vi "Digital display.vi"() -> ()   [LabVIEW 2019]
uses:
  <vilib>/addons/Modulation/Analog/controls/Complex Data Waveform.ctl
  <vilib>/measure/madcrms.llb/Averaged DC-RMS for 1 Chan.vi
  <vilib>/addons/Modulation/niAMT.lvlib
  <vilib>/measure/NI_MAPro.lvlib
panel:
  out "Waveform Graph 5":waveform(dbl)(graph)
  out "Waveform Graph 4":waveform(dbl)(graph)
  out "Digital Waveform Graph 2":digitalwaveform(graph)
  out "Digital Waveform Graph":digitalwaveform(graph)
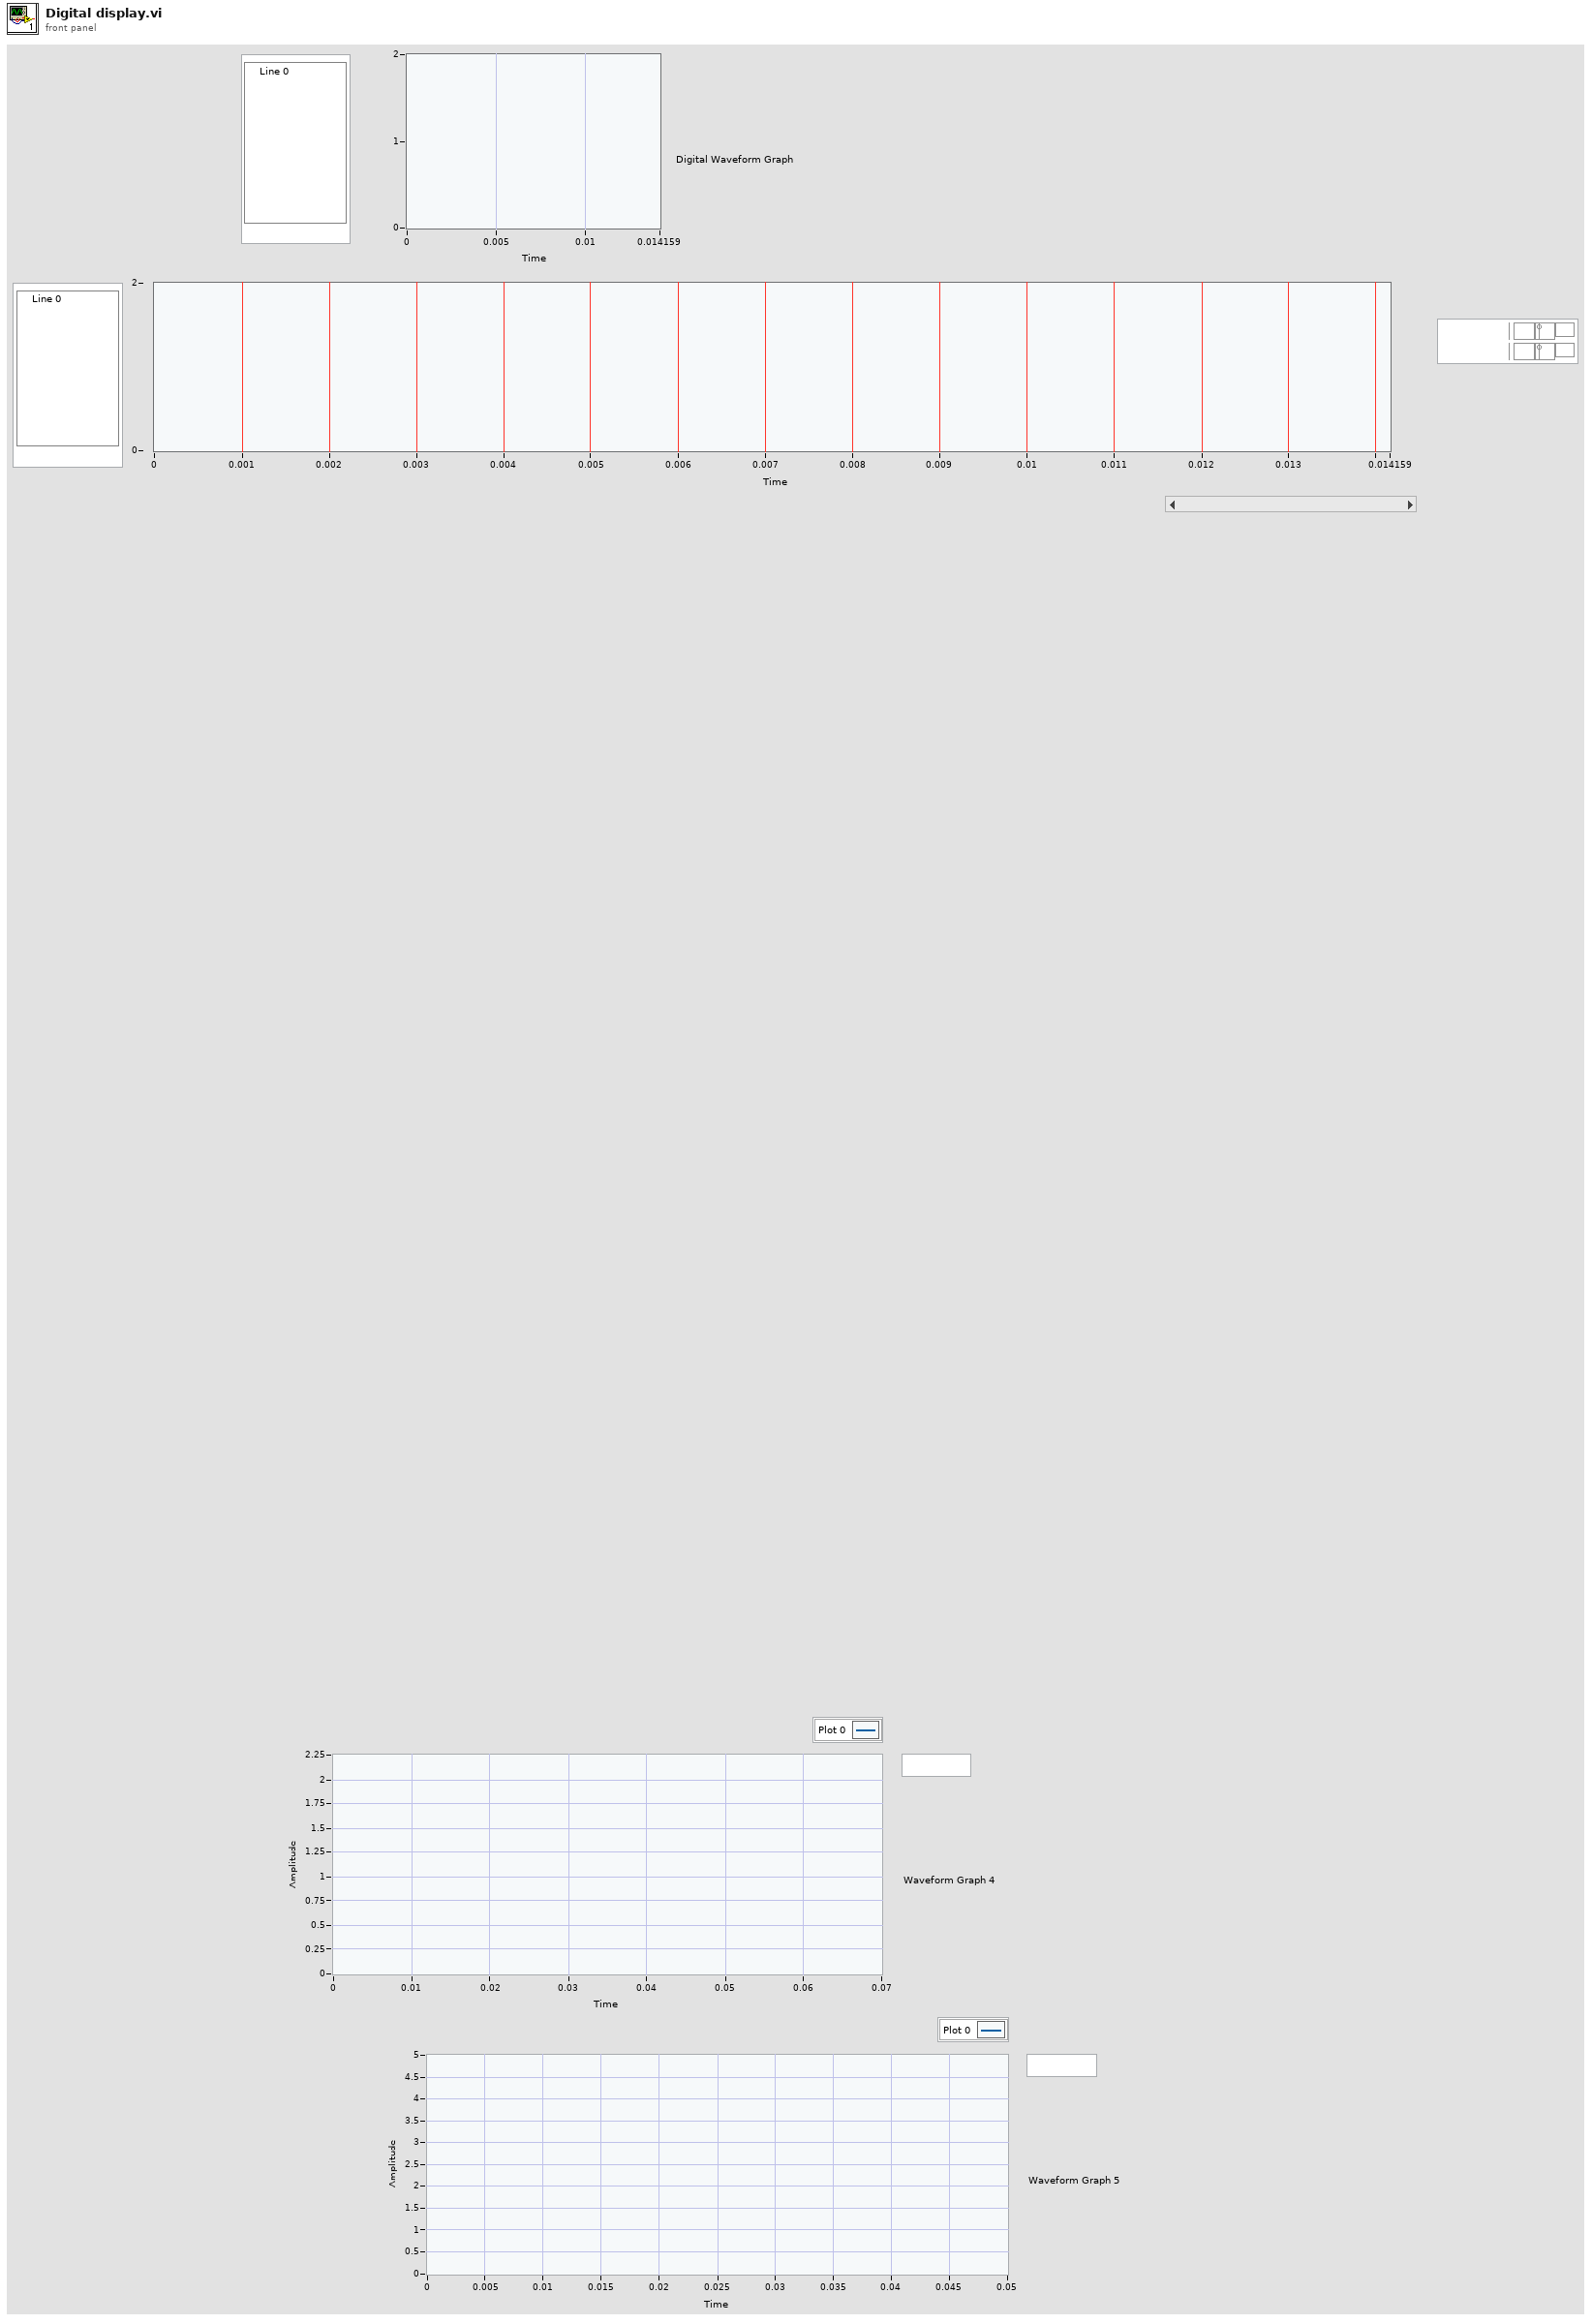
[diagram p1: front panel]
types:
  T1 = cluster{"window for DC":enum16{"Rectangular (none)", "Hanning", "Low side lobe"}, "output function":enum16{"DC only", "RMS only", "DC and RMS"}, "window for RMS":enum16{"Rectangular (none)", "Hanning", "Low side lobe"}, "exp. time constant":dbl, "Ignore input start time":bool}
  T2 = typedef "niAMT.lvlib/Complex Data Waveform.ctl" = cluster{"t0":dbl, "dt":dbl, "Y":cdb[]}
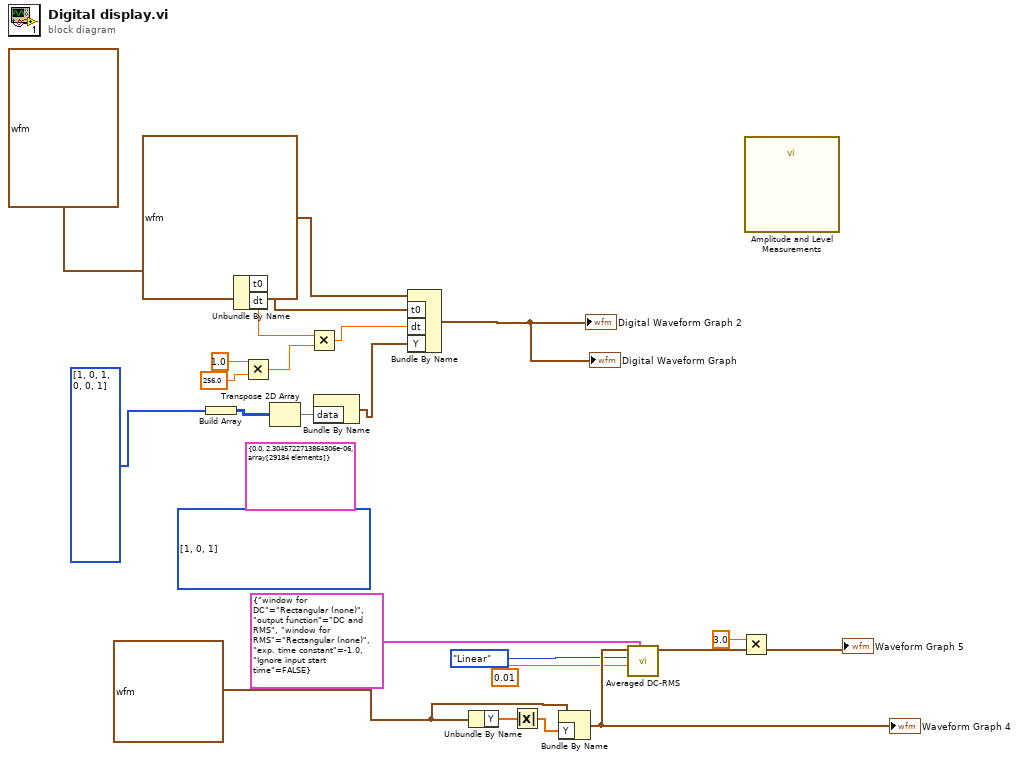
[diagram p0: block diagram]
diagram:
  w9 = waveform(dbl) {"t0"=timestamp(0 s since 1904-01-01), "dt"=2.3045722713864306e-06, "Y"=array[29568 elements]} ("Waveform out")
  (unwired) T2 {"t0"=0.0, "dt"=2.3045722713864306e-06, "Y"=array[29184 elements]} ("recovered complex waveform")
  (unwired) u8[][] [[1], [0], [1]] ("data")
  n1 = Build Array(i32[] [1, 0, 1, 0, 0, 1]) -> (w23:i32[][])
  n2 = Unbundle By Name(waveform(dbl) {"t0"=timestamp(6.868436578171096 s since 1904-01-01), "dt"=9.218289085545723e-06, "Y"=array[7296 elements]} ("Waveform")) -> ("t0"=w18:timestamp, "dt"=w17:dbl)
  n3 = Multiply(x=1.0 ("y"), y=256.0) -> (x*y=w13:dbl)
  n4 = Transpose 2D Array(2D array=w23) -> (transposed array=w21:i32[][])
  n5 = Multiply(x=w17, y=w13) -> (x*y=w16:dbl)
  n6 = Bundle By Name("data"=w21) -> (w20:digitaldata)  [unwired: 1 in]
  n7 = Bundle By Name(cluster=digitalwaveform {"t0"=timestamp(0 s since 1904-01-01), "dt"=1.0, "Y"={"transitions"=[], "data"=[]}} ("waveform"), "t0"=w18, "dt"=w16, "Y"=w20) -> (→"Digital Waveform Graph" →"Digital Waveform Graph 2":digitalwaveform)
  n8 = Unbundle By Name(w9) -> ("Y"=w10:dbl[])
  n9 = Absolute Value(x=w10) -> (abs(x)=w8:dbl[])
  n10 = Bundle By Name(cluster=w9, "Y"=w8) -> (w7:waveform(dbl))
  "Waveform Graph 4" <- w7
  n11 = call-poly <vilib>:"Averaged DC-RMS.vi"("averaging control"=T1 {"window for DC"=enum."Rectangular (none)", "output function"=enum."DC and RMS", "window for RMS"=enum."Rectangular (none)", "exp. time constant"=-1.0, "Ignore input start time"=FALSE}, "averaging time"=0.01, "averaging type"=enum16{"Linear", "Exponential"}."Linear", "signal in"=w7) -> ("DC value waveform"=w6:waveform(dbl))  [unwired: 3 in, 4 out]
  n12 = Multiply(x=3.0, y=w6) -> (x*y=→"Waveform Graph 5":waveform(dbl))
  n13 = call "Amplitude and Level Measurements"() -> ()  [unwired: 15 in, 1 out]
